vi "Build Channel Cluster Array.vi"() -> (3 "Channels out":cluster{"Channels":T1[]})   [LabVIEW 2023, in "Device Cluster - 1 Channel.lvclass"]
uses:
  Device Cluster - 1 Channel.lvclass
  Utilities/Channel.ctl
  Device Cluster - 1 Channel.lvclass/Device Cluster - 1 Channel.ctl
  Utilities/Utilities.lvlib
panel:
  in  "Channels in":cluster{"Channels":T1[]}
  in  "Chiller Cluster - 1 Channel.lvclass":refnum<class "Device Cluster - 1 Channel.lvclass">
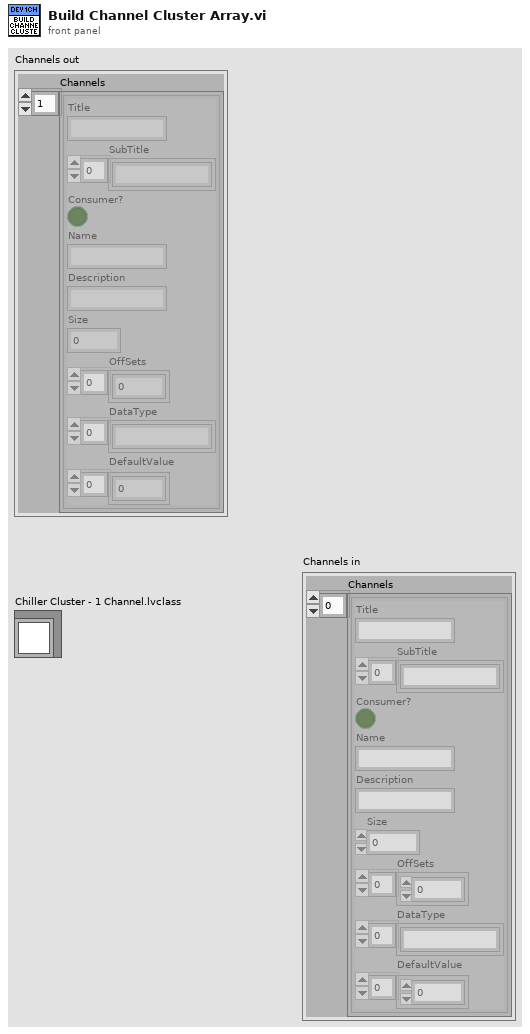
[diagram p1: front panel]
types:
  T1 = typedef "Utilities.lvlib/Channel.ctl" = cluster{"Title":string, "SubTitle":string[], "Consumer?":bool, "Name":string, "Description":string, "Size":i32, "OffSets":i32[], "DataType":string[], "DefaultValue":dbl[]}
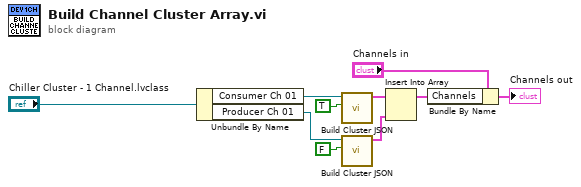
[diagram p0: block diagram]
diagram:
  n1 = Unbundle By Name("Chiller Cluster - 1 Channel.lvclass") -> ("Consumer Ch 01"=w3:refnum<k21>, "Producer Ch 01"=w4:refnum<k21>)
  n2 = call "Build Cluster JSON.vi"("Consumer?"=TRUE, "Cluster"=w3) -> ("Array"=w2:T1[])  [unwired: 9 in]
  n3 = call "Build Cluster JSON.vi"("Consumer?"=FALSE, "Cluster"=w4) -> ("Array"=w1:T1[])  [unwired: 9 in]
  n4 = Insert Into Array(array=w2, new element=w1) -> (w8:T1[])  [unwired: 1 in]
  n5 = Bundle By Name(cluster="Channels in", "Channels"=w8) -> (→"Channels out":cluster{"Channels":T1[]})
